vi "Dashboard Main.vi"() -> ()   [LabVIEW 2014]
uses:
  <vilib>/event_ctls.llb/eventvkey.ctl
  <vilib>/Utility/config.llb/NI_LVConfig.lvlib
  <vilib>/Rock Robotics/WPI/Dashboard/WPI_DashboardLogging Global.vi
  <vilib>/Utility/config.llb/Write Key (Boolean).vi
  <vilib>/Utility/config.llb/Write Key (String).vi
panel:
  out "Time":string
  out "Process?":bool
  in  "Listbox":i32(listbox)
  out "Progress":T1 {"Test Progress" scale=0.0..100.0}
  in  "Motor":cluster{"Value":dbl, "Enable":bool} {"Value" scale=-1.0..1.0 scale format="%#_3g"}
  in  "Test Slider":dbl(slide) scale=0.0..100.0 scale format="%#_3g"
  in  "On/Off":bool caption="Solenoid"
  in  "Test Name":u16(ring) items=["Select the test to run..."]
  in  "Rev/Fwd":cluster{"Forward":bool, "Reverse":bool}
  in  "Test Ring":u16(ring) items=["Monochrome", "Color"]
  in  "Test Tree":string(tree)
  in  "DB/String 9":string
  in  "DB/String 8":string
  in  "DB/String 7":string
  in  "DB/String 6":string
  in  "DB/String 5":string
  in  "DB/String 4":string
  in  "DB/String 3":string
  in  "DB/String 2":string
  in  "DB/String 1":string
  in  "DB/String 0":string
  in  "DB/Slider 0":dbl(slide) scale=0.0..5.0
  in  "DB/Slider 1":dbl(slide) scale=0.0..5.0
  in  "DB/Slider 2":dbl(slide) scale=0.0..5.0
  in  "DB/Slider 3":dbl(slide) scale=0.0..5.0
  out "DB/LED 3":bool
  out "DB/LED 2":bool
  out "DB/LED 1":bool
  out "DB/LED 0":bool
  in  "DB/Button 3":bool
  in  "DB/Button 2":bool
  in  "DB/Button 1":bool
  in  "DB/Button 0":bool caption="New Name"
  in  "TCP":refnum<k5>
  in  "Rec Mode":enum32{"Stop", "Record", "Playback"}(radio)
  in  "Vision":u16(ring) items=["Camera Off", "USB Camera SW", "USB Camera HW", "IP Camera"]
  out "Camera IP":string
  out "Image Message":string="Timeout in Camera Communications"
  in  "Dashboard Tab":T2(tab)
  out "Gyro":dbl(knob) scale=0.0..360.0
  out "JS1 Z 3":dbl(slide) scale=-1.0..1.0 scale format="%#_2e"
  out "JS1 Graph 3":cluster{"X":dbl, "Y":dbl}[](graph)
  out "JS1 Buttons 3":T3
  out "JS1 Z 2":dbl(slide) scale=-1.0..1.0 scale format="%#_2e"
  out "JS1 Graph 2":cluster{"X":dbl, "Y":dbl}[](graph)
  out "JS1 Buttons 2":T3
  in  "Dropdown":u8(ring) items=["Red 1", "Red 2", "Red 3", "Blue 1", "Blue 2", "Blue 3"]
  out "MotorChart R":cluster{"Numeric":dbl, "Numeric":dbl}(graph)
  out "MotorChart L":T4(graph)
  out "MotorSliders R":cluster{"MotorSlide1":dbl, "MotorSlide2":dbl} {"MotorSlide2" scale=-1.0..1.0 scale format="%#_2e"; "MotorSlide1" scale=-1.0..1.0 scale format="%#_2e"}
  out "MotorSliders L":T5 {"MotorSlide4 2" scale=0.0..14.0 scale format="%#_2e"; "MotorSlide2" scale=-1.0..1.0 scale format="%#_2e"; "MotorSlide1" scale=-1.0..1.0 scale format="%#_2e"}
  out "JS1 Z":dbl(slide) scale=-1.0..1.0 scale format="%#_2e"
  out "JS1 Graph":cluster{"X":dbl, "Y":dbl}[](graph)
  out "JS1 Buttons":T3
  out "Robot IP":string
  out "Dash Milliseconds Per Iteration":u32(knob) scale=250.0..500.0
  out "Dash Iterations Per Second":u32(knob)=4
  out "Main Milliseconds Per Iteration":u32(knob) scale=20.0..50.0
  out "CAN":T6 {"% Bus Utilization" format="%#_g%"}
  out "CAN BUS %":sgl(slide) scale=0.0..100.0
  out "CPU %":sgl(slide) scale=0.0..100.0
  out "RAM Usage":u32(slide) scale=0.0..100.0
  out "Storage":T7
  out "CPU Utilization":T8 {"CPU % ISR" format="%#_g%"; "CPU % Time Crit" format="%#_g%"; "CPU % Timed Str" format="%#_g%"; "CPU % High" format="%#_g%"; "CPU % Above" format="%#_g%"; "CPU % Normal" format="%#_g%"; "CPU % Low" format="%#_g%"}
  out "Main Iterations Per Second":u32(knob)=50
  in  "export stat":bool
  out "Stats":sgl[](graph)
  in  "clear stat":bool
  out "Tree":string(tree)
  out "Camera Image":T9(plugin-control)
  out "Boolean":bool
  # "Joysticks"
  # "SubStates"
  # "Drive & Battery"
  # "Encoders"
  # "Left"
  # "Front"
  # "Right"
  # "Battery"
  # "Chart of the below shown  data over time on next tab"
  # "Robot Metrics"
  # "Code Statistics"
  # "IPS"
  # "mSPI"
  # "IPS"
  # "mSPI"
  # "See the below driver station for\ngraphs of CPU%"
  # "Optimal Speeds (Statistics)\n\nMain mSPI = 20 ms\nMain IPS  = 50 iterations\n\nDash mSPI = 250 ms\nDash IPS  = 4 iterations\n\nKey\n\nmSPI - miliseconds per iteration\nIPS - iterations per second"
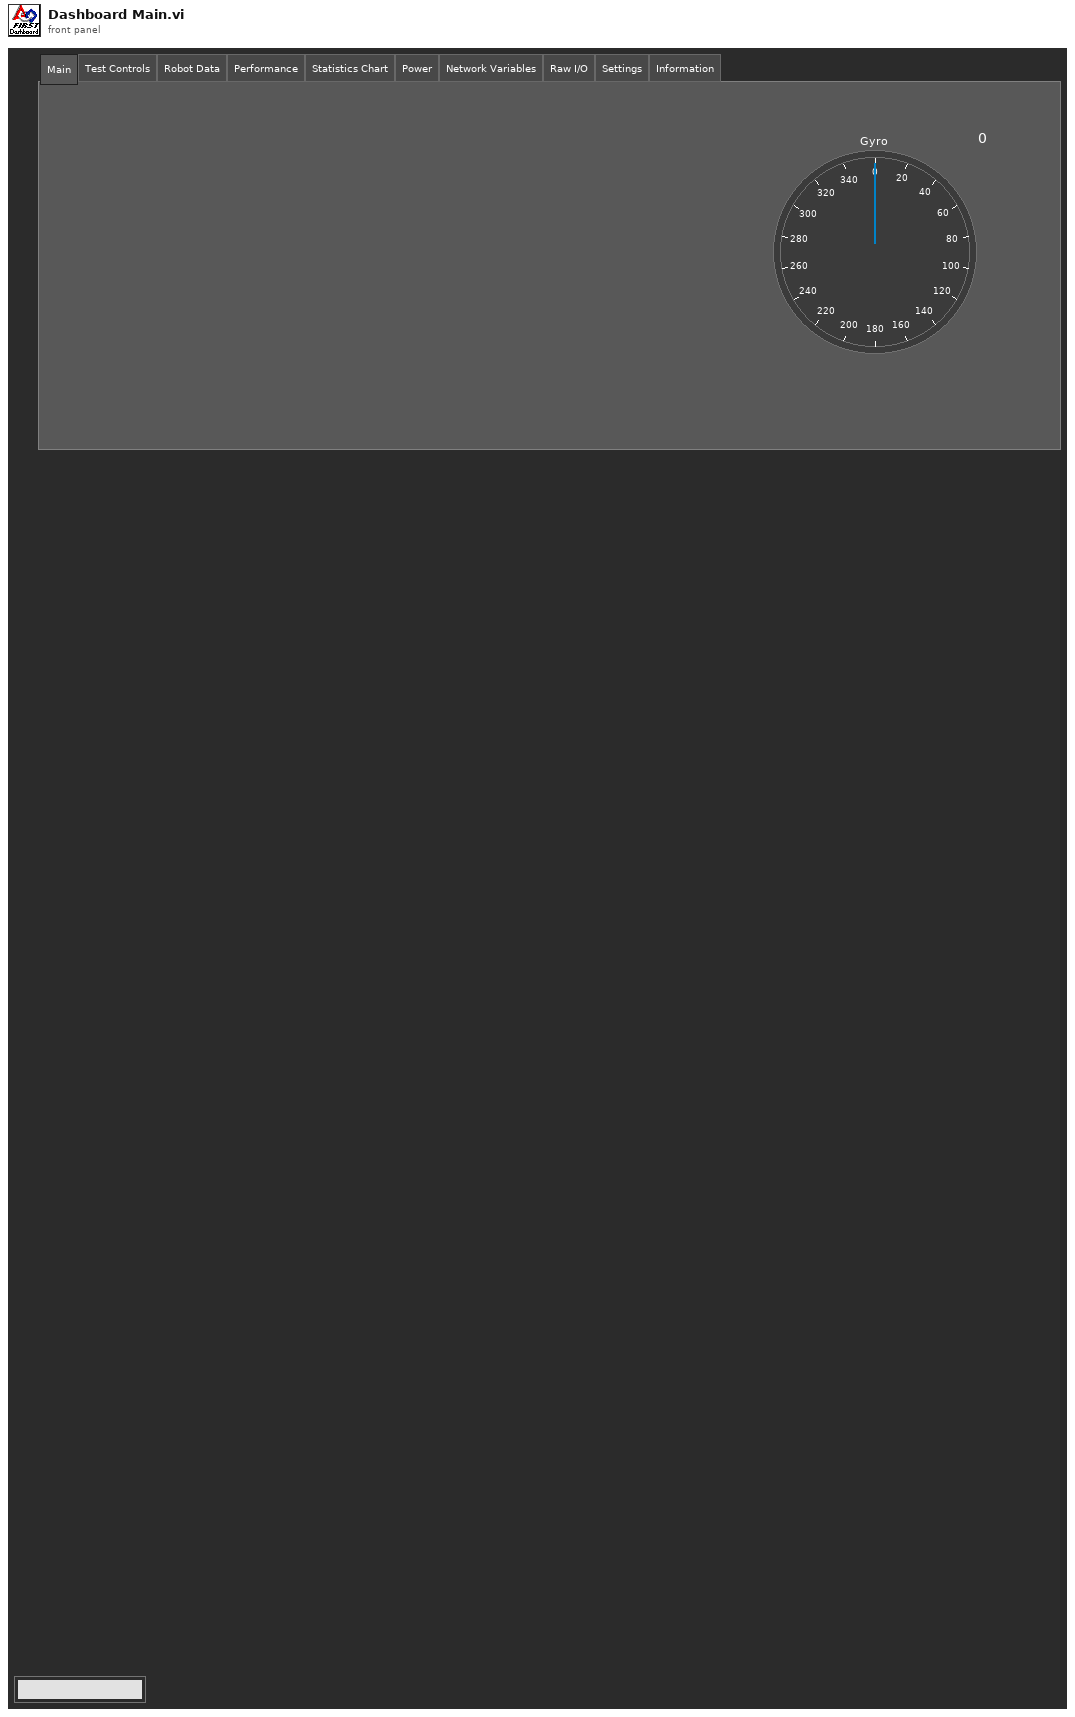
[diagram p1: front panel]
types:
  T1 = cluster{"Test Progress":u8, "Test Progress Text":string}
  T2 = enum32{"Main", "Test Controls", "Robot Data", "Performance", "Statistics Chart", "Power", "Network Variables", "Raw I/O", "Settings", "Information"}
  T3 = cluster{bool, bool, bool, bool, bool, bool, bool, bool, bool, bool, bool, bool}
  T4 = cluster{"Numeric":dbl, "Numeric":dbl, "Battery V":dbl}
  T5 = cluster{"MotorSlide1":dbl, "MotorSlide2":dbl, "MotorSlide4 2":dbl}
  T6 = cluster{"% Bus Utilization":sgl, "Bus Off Cnt":u32, "TX_FIFO Full Cnt":u32, "Receive Error Cnt":u8, "Transmit Error Cnt":u8}
  T7 = cluster{"Disk Free":u64, "RAM Block":u32, "RAM free":u32}
  T8 = cluster{"CPU % ISR":sgl, "CPU % Time Crit":sgl, "CPU % Timed Str":sgl, "CPU % High":sgl, "CPU % Above":sgl, "CPU % Normal":sgl, "CPU % Low":sgl}
  T9 = typedef "IMAQ Image.ctl" = refnum<image>
  T10 = enum32{"Drive", "Basic", "Custom", "Test", "Checklist", "Variables"}
  T11 = cluster{"Camera Image":refnum<vi>, "Dashboard Tab":refnum<vi>, "Boolean":refnum<vi>, "Vision":refnum<vi>, "Rec Mode":refnum<vi>, "Test Slider":refnum<vi>, "On/Off ":refnum<vi>, "Test Ring":refnum<vi>, "Rev/Fwd":refnum<vi>, "Test Name":refnum<vi>, "Motor":refnum<vi>, "Progress":refnum<vi>, "CheckList":refnum<vi>, "Tree":refnum<vi>, "Test Tree":refnum<vi>}
  T12 = cluster{"Error Strings":string, "Disable Counts":cluster{u16, u16}, "Rail Faults":cluster{u16, u16, u16}, "Robot IP":string, "DB Mode":u8, "Event Info":cluster{"Name":string, "Type":u8, "Number":u16, "Replay":u8}, "Camera Addr":string}
  T13 = cluster{"Storage":cluster{"Disk Free":u64, "RAM Block":u32, "RAM free":u32}, "CPU Utilization":cluster{"CPU % ISR":sgl, "CPU % Time Crit":sgl, "CPU % Timed Str":sgl, "CPU % High":sgl, "CPU % Above":sgl, "CPU % Normal":sgl, "CPU % Low":sgl}, "CAN":cluster{"% Bus Utilization":sgl, "Bus Off Cnt":u32, "TX_FIFO Full Cnt":u32, "Receive Error Cnt":u8, "Transmit Error Cnt":u8}, "HID":cluster{"HID Outputs":u32, "Rumble Low":u16, "Rumble High":u16}[]}
  T14 = cluster{"Status bits":cluster{"Test Mode":bool, "Autonomous":bool, "Enabled":bool, "Code Start":bool, "Brownout":bool, "Reserved 2":bool, "Reserved 3":bool, "E-Stop":bool}, "Code Trace":cluster{"Disabled":bool, "TeleOp":bool, "Auto":bool, "Test":bool}, "Controller Type":enum16{"unknown", "cRIO", "roboRio"}, "Code?":enum16{"unknown", "noCode", "code"}, "Battery V":dbl}
  T15 = cluster{"Control Bits":cluster{"TestMode":bool, "Autonomous":bool, "Enabled":bool, "FMS Present":bool, bool, bool, bool, "E-Stop":bool}, "Team Station ":u8, "Countdown":sgl, "Joystick Values":cluster{"Axes":dbl[], "Buttons":bool[], "POVs":i16[]}[]}
  T16 = enum8{"Tele-Op Disabled", "Tele-Op Enabled", "Auto Disabled", "Auto Enabled", "Test Disabled", "Test Enabled", "Disconnected", "No Code", "E-Stop"}
  T17 = cluster{"Axes":dbl[], "Buttons":bool[], "POVs":i16[]}[]
  T18 = cluster{"Axes":dbl[], "Buttons":bool[], "POVs":i16[]}
  T19 = cluster{"Buttons[0]":bool, "Buttons[1]":bool, "Buttons[2]":bool, "Buttons[3]":bool, "Buttons[4]":bool, "Buttons[5]":bool, "Buttons[6]":bool, "Buttons[7]":bool, "Buttons[8]":bool, "Buttons[9]":bool, "Buttons[10]":bool, "Buttons[11]":bool}
  T20 = typedef "Image Type" = u32
  T21 = typedef "WPI_CameraSettings Read MJPG.ctl" = cluster{"fps":i32, "compression":i32, "Image Size":T22}
  T22 = typedef "WPI_CameraImageSize.ctl" = enum16{"640x480", "320x240", "160x120", "Custom"}
  T23 = cluster{"Operation":enum16{"Update", "Clear"}, "Color Box":u32}[]
  T24 = typedef "eventvkey.ctl" = enum16{"ASCII", "Enter", "Return", "Shift", "Ctrl", "Alt", "Cmd", "Opt", "Caps", "NumLock", "Clear", "Break", "Up", "Down", "Left", "Right", "Insert", "Delete", "Home", "End", "PageUp", "PageDown", "Escape", "Help", "Pause", "ScrollLock", "F1", "F2", "F3", "F4", "F5", "F6", "F7", "F8", "F9", "F10", "F11", "F12", "F13", "F14", "F15", "F16", "F17", "F18", "F19", "F20", "F21", "F22", "F23", "F24", "Play", "VolumeUp", "VolumeDown", "Mute", "Two Byte Char"}
  T25 = cluster{"Image Size":bool, "Image Type":bool, "Pixel Value":bool, "ROI Information":bool, "Zoom Factor":bool}
  T26 = enum8{"Enabled", "Disabled", "Disabled and Grayed Out"}
  T27 = typedef "NI_LVConfig.lvlib/Config Data RefNum.ctl" = refnum<k1>
  T28 = cluster{"Operation":enum16{"Update", "Clear"}, "Color Box":u32}
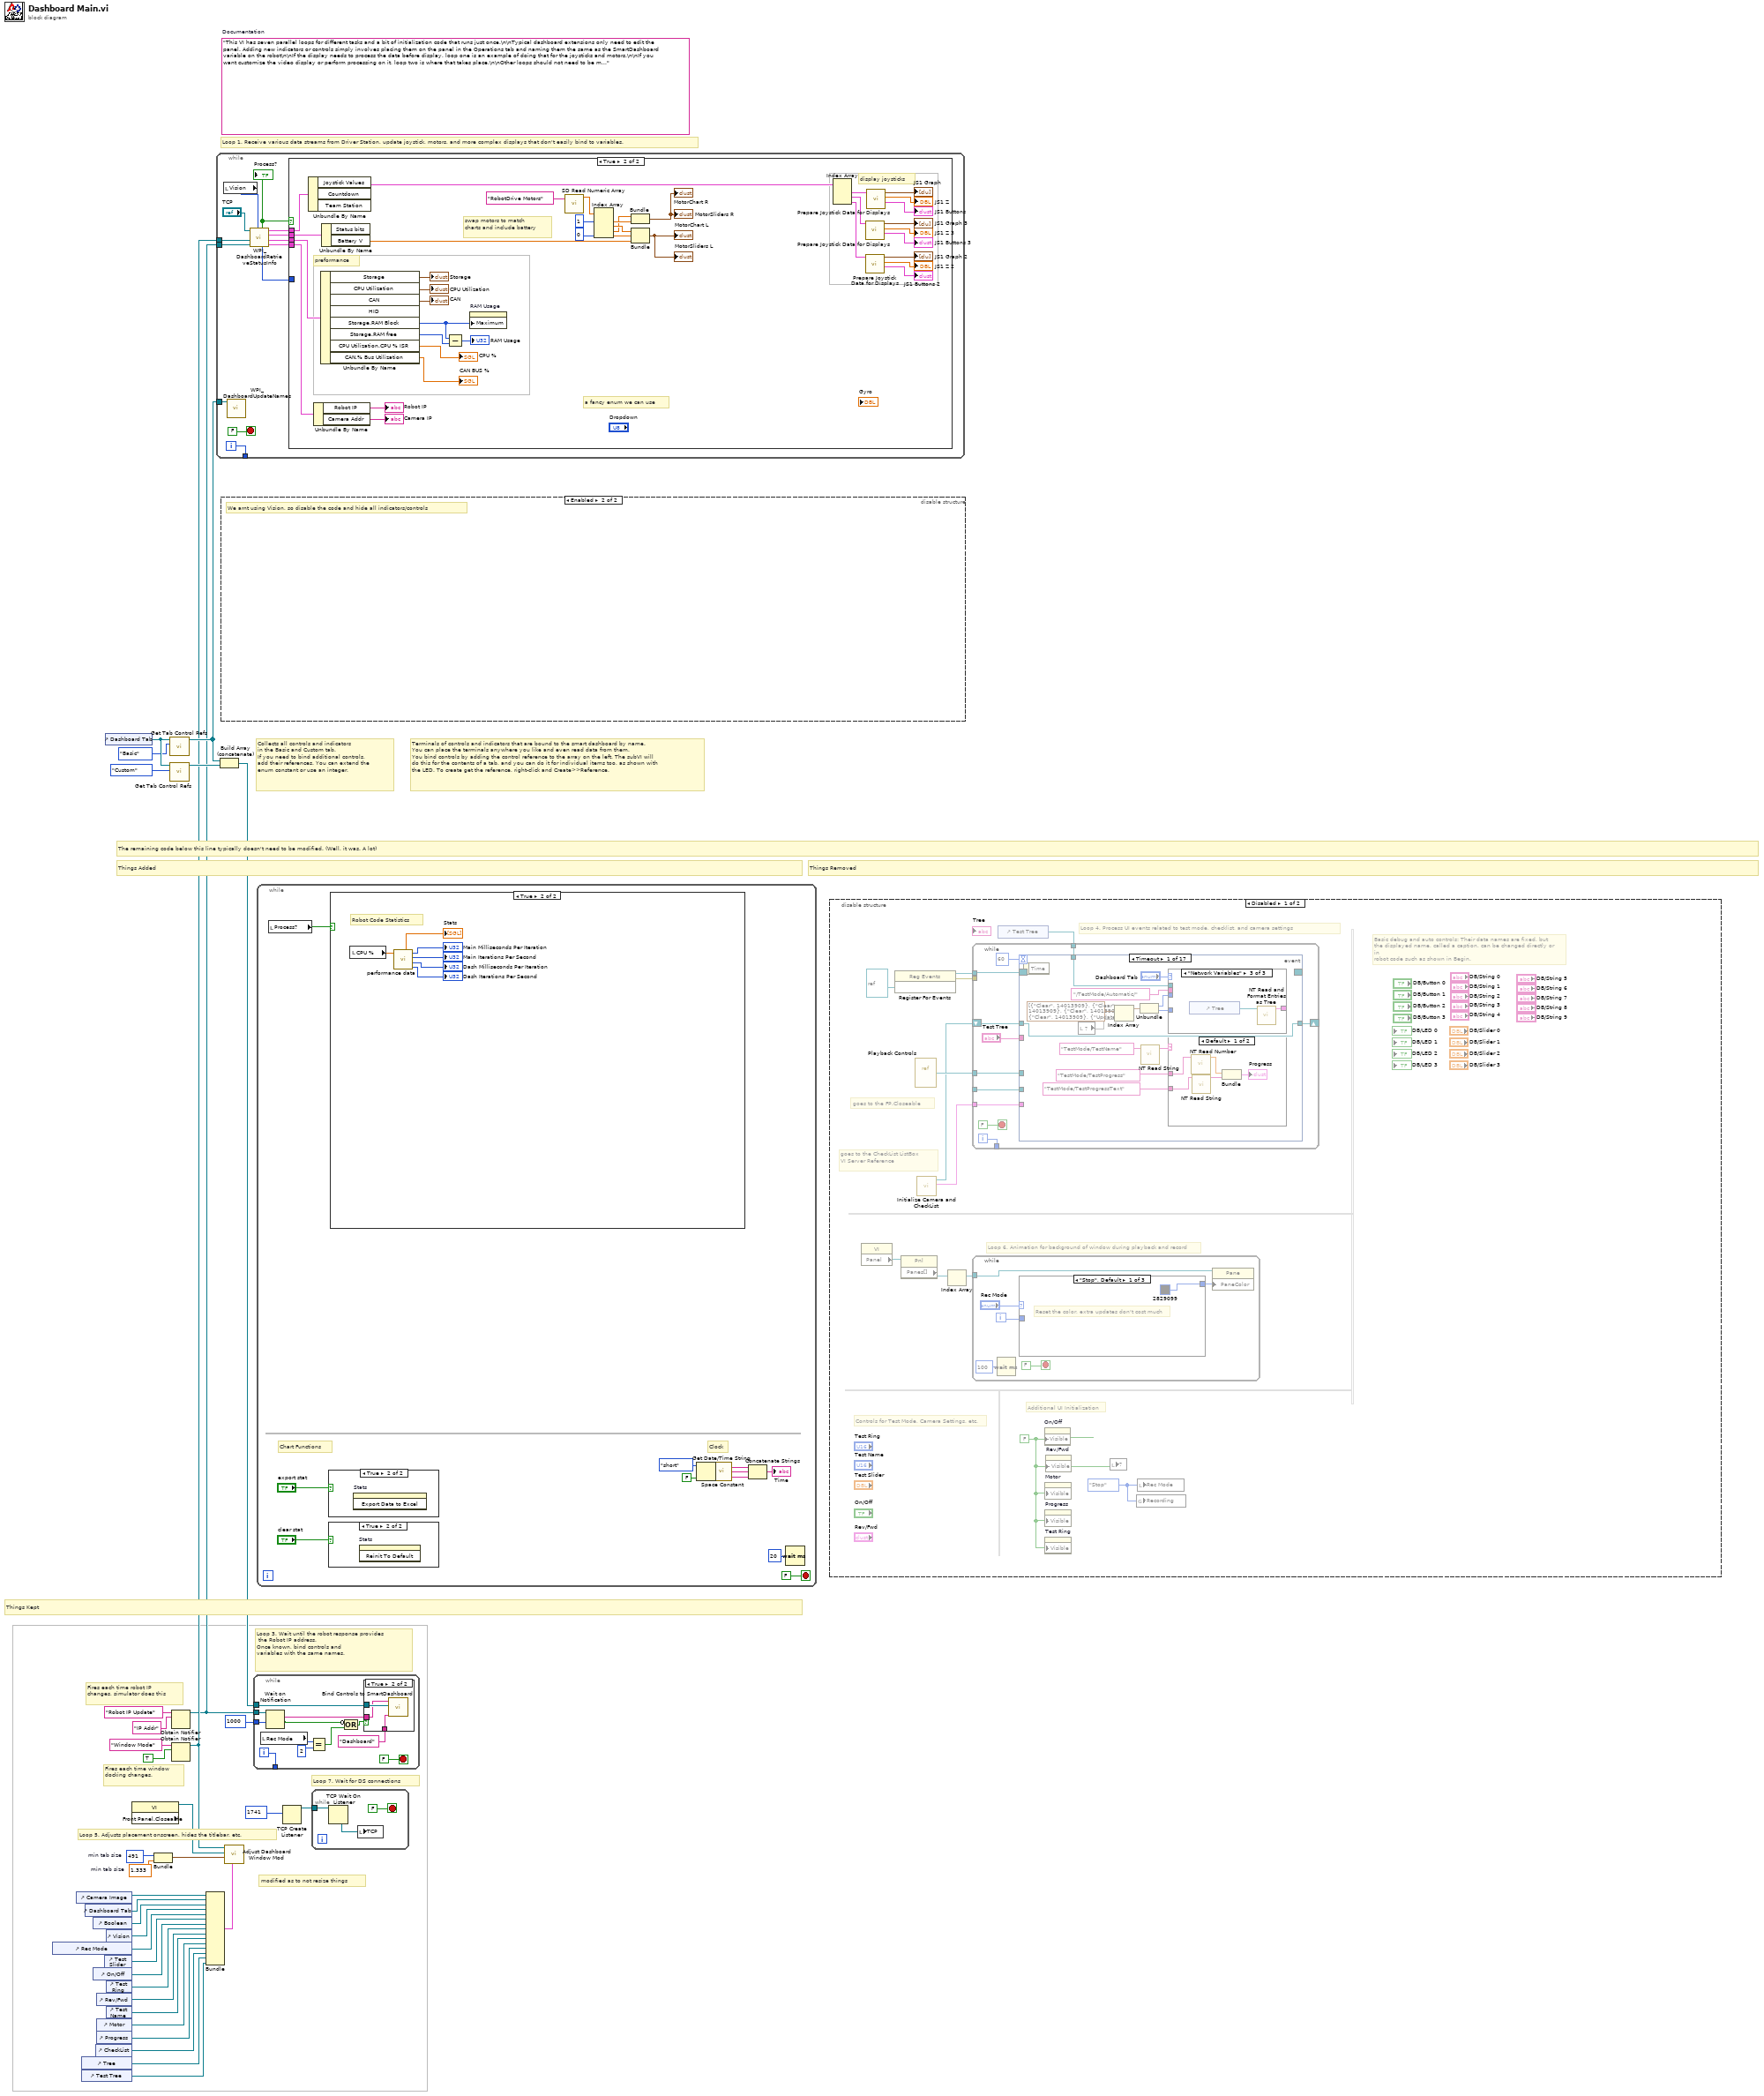
[diagram p0: block diagram]
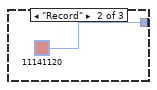
[diagram p5: hidden frame]
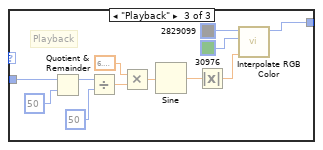
[diagram p6: hidden frame]
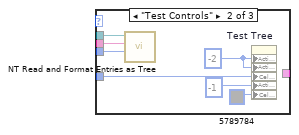
[diagram p8: hidden frame]
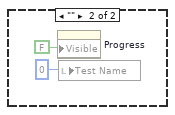
[diagram p9: hidden frame]
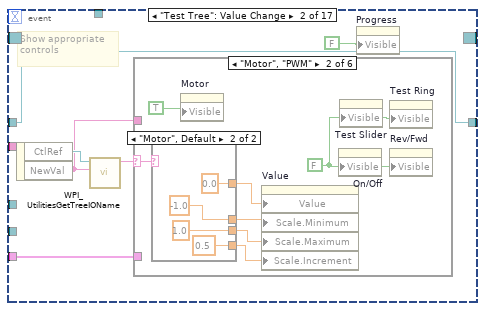
[diagram p10: hidden frame]
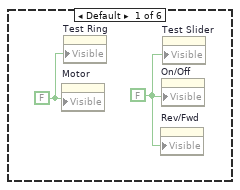
[diagram p11: hidden frame]
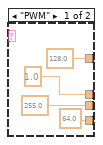
[diagram p12: hidden frame]
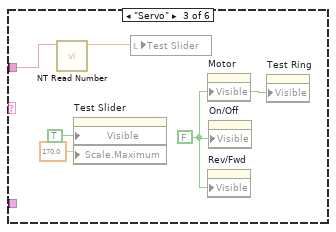
[diagram p13: hidden frame]
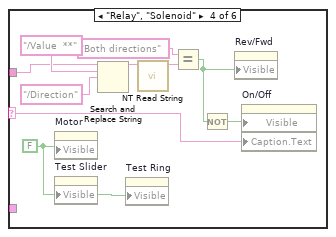
[diagram p14: hidden frame]
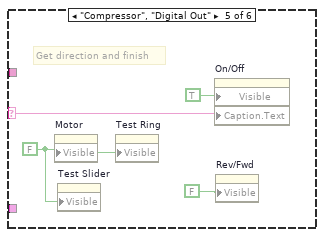
[diagram p15: hidden frame]
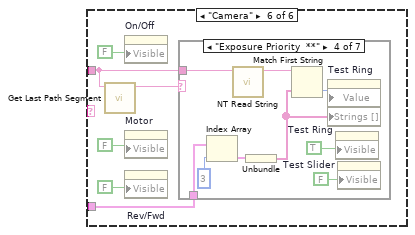
[diagram p16: hidden frame]
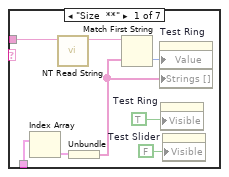
[diagram p17: hidden frame]
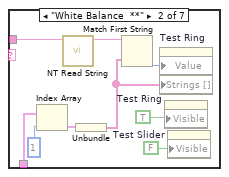
[diagram p18: hidden frame]
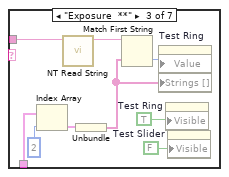
[diagram p19: hidden frame]
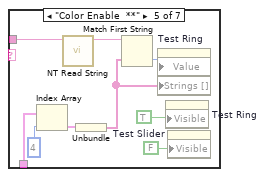
[diagram p20: hidden frame]
diagram:
  w24 = 491  # min tab size
  w23 = 1.333  # min tab size
  (unwired) "This VI has seven parallel loops for different tasks and a bit of initialization code that runs just once.\n\nTypical dashboard extensions only need to edit the panel. Adding new indicators or controls simply involves placing them on the panel in the Operations tab and naming them the same as the SmartDashboard variable on the robot\n\nIf the display needs to process the data before display, loop one is an example of doing that for the joysticks and motors.\n\nIf you want customize the video display or perform processing on it, loop two is where that takes place.\n\nOther loops should not need to be modified. They are pretty standard, and document the task they perform."  # Documentation
  # "modified as to not resize things"
  # "Things Kept"
  # "Things Added"
  # "Things Removed"
  # "Loop 7. Wait for DS connections"
  # "Fires each time robot IP\nchanges, simulator does this"
  # "Fires each time window\ndocking changes."
  # "Collects all controls and indicators\nin the Basic and Custom tab.\nIf you need to bind additional controls,\nadd their references. You can extend the\nenum constant or use an integer."
  # "The remaining code below this line typically doesn't need to be modified. (Well, it was. A lot)"
  # "Terminals of controls and indicators that are bound to the smart dashboard by name.\nYou can place the terminals anywhere you like and even read data from them.\nYou bind controls by adding the control reference to the array on the left. The subVI will\ndo this for the contents of a tab, and you can do it for individual items too, as shown with\nthe LED. To create get the reference, right-click and Create>>Reference."
  # "Loop 3. Wait until the robot response provides\n the Robot IP address.\nOnce known, bind controls and\nvariables with the same names."
  # "Loop 5. Adjusts placement onscreen, hides the titlebar, etc."
  # "Loop 1. Receive various data streams from Driver Station, update joystick, motors, and more complex displays that don't easily bind to variables."
  n1 = control-ref of="Rec Mode"() -> (w15:refnum<vi>)
  n2 = control-ref of="Camera Image"() -> (w27:refnum<vi>)
  n3 = control-ref of="Tree"() -> (w19:refnum<vi>)
  n4 = control-ref of="Test Tree"() -> (w18:refnum<vi>)
  n5 = control-ref of="Dashboard Tab"() -> (w26:refnum<vi>)
  n6 = control-ref of="Boolean"() -> (w22:refnum<vi>)
  n7 = control-ref of="On/Off"() -> (w13:refnum<vi>)
  n8 = control-ref of="CheckList"() -> (w6:refnum<vi>)
  n9 = control-ref of="Rev/Fwd"() -> (w11:refnum<vi>)
  n10 = control-ref of="Motor"() -> (w16:refnum<vi>)
  n11 = control-ref of="Progress"() -> (w10:refnum<vi>)
  n12 = control-ref of="Test Slider"() -> (w14:refnum<vi>)
  n13 = control-ref of="Dashboard Tab"() -> (w30:refnum<vi>)
  n14 = control-ref of="Vision"() -> (w25:refnum<vi>)
  n15 = control-ref of="Test Ring"() -> (w12:refnum<vi>)
  n16 = control-ref of="Test Name"() -> (w17:refnum<vi>)
  n17 = property class="VI" props=["Front Panel.Closeable"]() -> (reference out=w3:refnum<vi>)  [unwired: 2 in, 2 out]
  n18 = Bundle("min tab size"=w24, "min tab size"=w23) -> (w4:cluster{"min tab size":i32, "min tab size":dbl})  [unwired: 1 in]
  n19 = call <vilib>:"Get Tab Control Refs.vi"("Page Index"=T10."Basic" ("Dashboard Tab"), "TabControl in"=w30) -> ("ControlsOnPage"=w9:refnum<vi>[])  [unwired: 9 in]
  n20 = call <vilib>:"Get Tab Control Refs.vi"("Page Index"=T10."Custom" ("Dashboard Tab"), "TabControl in"=w30) -> ("ControlsOnPage"=w29:refnum<vi>[])  [unwired: 9 in]
  n21 = Obtain Notifier(name (unnamed)="Robot IP Update", notification data type="IP Addr" ("name (unnamed)")) -> (notifier out=w1:refnum<notifier>)  [unwired: 2 in, 2 out]
  n22 = Obtain Notifier(name (unnamed)="Window Mode", notification data type=TRUE) -> (notifier out=w2:refnum<notifier>)  [unwired: 2 in, 2 out]
  n23 = Bundle("Camera Image"=w27, "Dashboard Tab"=w26, "Boolean"=w22, "Vision"=w25, "Rec Mode"=w15, "Test Slider"=w14, "On/Off"=w13, "Test Ring"=w12, "Rev/Fwd"=w11, "Test Name"=w17, "Motor"=w16, "Progress"=w10, "CheckList"=w6, "Tree"=w19, "Test Tree"=w18) -> (w5:T11)  [unwired: 1 in]
  n24 = while {
    tunnel: [w47] -> _
    tunnel: w1 -> [w41]
    tunnel: w9 -> [w40]
    tunnel: w2 -> [w36]
    i -> [w47]
    stop <- FALSE stop-if-true
    n25 = local read "Vision"() -> (w38:u16)
    n26 = call <vilib>:"WPI_DashboardUpdateNames.vi"("Controls on Tab"=w40) -> ()  [unwired: 11 in]
    n27 = call <vilib>:"WPI_DashboardRetrieveStatusInfo.vi"("Vision"=w38, "Binding Refnum"=w41, "Window Mode Notifier"=w36, "TCP Cnx"="TCP") -> ("Power and Errors"=w42:T12, "Robot Metrics"=w45:T13, "Status Info"=w46:T14, "Control Info"=w43:T15, "Robot Mode"=w39:T16, "Process?"=w44:bool)  [unwired: 2 in]
    "Process?" <- w44
    n28 = case shown="True" w44 {
      tunnel: w46 -> [_ w86]
      tunnel: w45 -> [_ w85]
      tunnel: w43 -> [_ w84]
      tunnel: w42 -> [_ w83]
      tunnel: w39 -> [_ _]
      frame False {
      }
      frame True {
        # "preformance"
        # "display joysticks"
        # "a fancy enum we can use"
        # "swap motors to match\ncharts and include battery"
        n29 = Unbundle By Name(w84) -> ("Joystick Values"=w73:T17)  [unwired: 2 out]
        n30 = Unbundle By Name(w83) -> ("Robot IP"=→"Robot IP":string, "Camera Addr"=→"Camera IP":string)
        n31 = Unbundle By Name(w85) -> ("Storage"=→"Storage":T7, "CPU Utilization"=→"CPU Utilization":T8, "CAN"=→"CAN":T6, "Storage.RAM Block"=w52:u32, "Storage.RAM free"=w51:u32, "CPU Utilization.CPU % ISR"=→"CPU %":sgl, "CAN.% Bus Utilization"=→"CAN BUS %":sgl)  [unwired: 1 out]
        n32 = Unbundle By Name(w86) -> ("Battery V"=w74:dbl)  [unwired: 1 out]
        n33 = Subtract(x=w52, y=w51) -> (x-y=→"RAM Usage":u32)
        n34 = property on="RAM Usage" class="Slide (strict)"("Maximum"=w52) -> ()  [unwired: 2 in, 2 out]
        n35 = call <vilib>:"SD Read Numeric Array.vi"("Name"="RobotDrive Motors") -> ("Numeric Array"=w76:dbl[])  [unwired: 8 in, 2 out]
        n36 = Index Array(array=w76, index #1=1, index #4=0) -> (element #1=w78:dbl, element #2=w79:dbl, element #3=w77:dbl, element #4=w82:dbl)  [unwired: 2 in]
        n37 = Bundle("Numeric"=w77, "Numeric"=w78) -> (→"MotorSliders R" →"MotorChart R":cluster{"Numeric":dbl, "Numeric":dbl})  [unwired: 1 in]
        n38 = Bundle("Numeric"=w79, "Numeric"=w82, "Battery V"=w74) -> (→"MotorSliders L" →"MotorChart L":T4)  [unwired: 1 in]
        n39 = Index Array(array=w73) -> (element #1=w72:T18, element #2=w70:T18, element #3=w66:T18)  [unwired: 3 in]
        n40 = call "Prepare Joystick Data for Displays.vi"("Joystick Values"=w70) -> ("Buttons"=→"JS1 Buttons 3":T19, "Z Axis"=→"JS1 Z 3":dbl, "Cartesian Data"=→"JS1 Graph 3":cluster{"X axis":dbl, "X axis":dbl}[])  [unwired: 8 in]
        n41 = call "Prepare Joystick Data for Displays.vi"("Joystick Values"=w66) -> ("Buttons"=→"JS1 Buttons 2":T19, "Z Axis"=→"JS1 Z 2":dbl, "Cartesian Data"=→"JS1 Graph 2":cluster{"X axis":dbl, "X axis":dbl}[])  [unwired: 8 in]
        n42 = call "Prepare Joystick Data for Displays.vi"("Joystick Values"=w72) -> ("Buttons"=→"JS1 Buttons":T19, "Z Axis"=→"JS1 Z":dbl, "Cartesian Data"=→"JS1 Graph":cluster{"X axis":dbl, "X axis":dbl}[])  [unwired: 8 in]
      }
    }
  }
  n43 = Build Array (concatenate)(w9, w29) -> (w28:refnum<vi>[])
  n44 = disable-structure shown="Enabled" {
    frame Disabled {
      w89 = T20 4 items=["Grayscale (U8)", "Grayscale (I16)", "Grayscale (SGL)", "Complex (CSG)", "RGB (U32)", "HSL (U32)", "RGB (U64)"] ("Image Type")
      # "unwired controls/indicators from below that orange line :P"
      # "Loop 2. Receive camera images from Robot, update Mbps, fps, and do any processing or display"
      n45 = call "IMAQ Create"("Image Name"="Dashboard Image", "Image Type"=w89) -> ("New Image"=w87:T9, "error out"=w88:errorcluster)  [unwired: 2 in, 1 out]
      n46 = while {
        tunnel: w87 -> [w99]
        tunnel: w88 -> [_]
        tunnel: [w100] -> _
        i -> [w100]
        stop <- FALSE stop-if-true
        # "Optionally read the DB image,\nlog, or retrieve images from a\nlogged match"
        n47 = local read "Rec Mode"() -> (w93:enum32{"Stop", "Record", "Playback"})
        n48 = local read "Camera IP"() -> (w91:string)
        n49 = call <vilib>:"WPI_CameraRead MJPG for Dashboard.vi"("Rec Mode"=w93, "Camera IP"=w91, "Camera Mode"="Vision", "Refnum in"=w99) -> ("Active"=w97:bool, "Refnum out"=w98:T9, "FPS"=w96:dbl, "Bandwidth (Mbps)"=w95:dbl, "Camera Settings"=w94:T21)  [unwired: 3 in]
        n50 = case shown="True" w97 {
          tunnel: w98 -> [_ w106]
          tunnel: w95 -> [_ w105]
          tunnel: w96 -> [_ w103]
          frame False {
            # "Sleep for 500ms"
            n51 = Wait Until Next ms Multiple(millisecond multiple=u32 500) -> ()  [unwired: 1 out]
          }
          frame True {
            # "Here is where you would annotate,\npossibly process, and display the image"
            # "Update Mbps LED"
            n52 = call "IMAQ Clear Overlay"("Image"=w106) -> ("error out"=w109:errorcluster, "Image Out"=→"Camera Image":T9)  [unwired: 2 in, 7 out]
            n53 = case shown="4, 5" w105 {
              tunnel: [u32 6618880 ("Color Box") u32 16776722 ("Color Box") u32 16716800 ("Color Box")] -> w107
              frame Default {
              }
              frame 4, 5 {
              }
              frame 6.. {
              }
            }
            n54 = Unbundle By Name(w109) -> ("status"=w110:bool)
            n55 = Bundle("Color Box"=w107, "Color Box"=w107) -> (w108:cluster{"Color Box":u32, "Color Box":u32})  [unwired: 1 out]
            n56 = property on="Image Message" class="Str"("Visible"=w110) -> ()  [unwired: 2 in, 2 out]
            n57 = Build Array(w108) -> ()  [unwired: 1 out]
          }
        }
      }
    }
    frame Enabled {
      # "We arnt using Vision, so disable the code and hide all indicators/controls"
    }
  }
  n58 = call "Adjust Dashboard Window Mod.vi"("Sizing Refnums"=w5, "Size Constraints"=w4, "VI"=w3, "Notifier in"=w2) -> ()  [unwired: 8 in]
  n59 = while {
    tunnel: w28 -> [w125]
    tunnel: w1 -> [w123]
    tunnel: [w121] -> _
    tunnel: u32 1000 ("milliseconds to wait") -> [w120]
    i -> [w121]
    stop <- FALSE stop-if-true
    n60 = local read "Rec Mode"() -> (w116:enum32{"Stop", "Record", "Playback"})
    n61 = Wait on Notification(notifier=w123, timeout in ms (-1)=w120) -> (notification=w122:string, timed out?=w118:bool)  [unwired: 2 in, 2 out]
    n62 = Equal?(x=w116, y=u16 2 ("Rec Mode")) -> (x = y?=w117:bool)
    n63 = Compound Arithmetic op=OR(invert w118, w117) -> (w119:bool)
    n64 = case shown="True" w119 {
      tunnel: w125 -> [_ w128]
      tunnel: w122 -> [_ w127]
      tunnel: "Dashboard" -> [_ w126]
      frame False {
      }
      frame True {
        n65 = call <vilib>:"Bind Controls to SmartDashboard.vi"("Client Name"=w126, "Bound Control Refs"=w128, "Server IP Address"=w127) -> ()  [unwired: 9 in]
      }
    }
  }
  n66 = while {
    stop <- FALSE stop-if-true
    # "Clock"
    # "Chart Functions"
    n67 = local read "Process?"() -> (w139:bool)
    n68 = case shown="True" "export stat" {
      frame False {
      }
      frame True {
        n69 = invoke on="Stats" class="WFChart (strict)" method="Export Data to Excel"() -> ()  [unwired: 3 in, 3 out]
      }
    }
    n70 = case shown="True" "clear stat" {
      frame False {
      }
      frame True {
        n71 = invoke on="Stats" class="WFChart (strict)" method="Reinit To Default"() -> ()  [unwired: 3 in, 3 out]
      }
    }
    n72 = case shown="True" w139 {
      frame False {
      }
      frame True {
        # "Robot Code Statistics"
        n73 = local read "CPU %"() -> (w144:sgl)
        n74 = call "performance data.vi"("CPU %"=w144) -> ("Dash IPS"=→"Dash Iterations Per Second":u32, "Dash mSPI"=→"Dash Milliseconds Per Iteration":u32, "Main IPS"=→"Main Iterations Per Second":u32, "Main mSPI"=→"Main Milliseconds Per Iteration":u32, "stats"=→"Stats":sgl[])  [unwired: 6 in]
      }
    }
    n75 = Get Date/Time String(date format (0)=enum16{"short", "long", "abbreviated"}."short", want seconds? (F)=FALSE) -> (date string=w131:string, time string=w132:string)  [unwired: 1 in]
    n76 = call <vilib>:"Space Constant.vi"() -> ("String"=w133:string)
    n77 = Concatenate Strings(w131, w133, w132) -> (→"Time":string)
    n78 = Wait (ms)(milliseconds to wait=u32 20) -> ()  [unwired: 1 out]
  }
  n79 = TCP Create Listener(10:u16 1741 ("timeout ms (25000)")) -> (3:w7:refnum<k5>)  [unwired: 4 in, 2 out]
  n80 = while {
    tunnel: w7 -> [w147]
    stop <- FALSE stop-if-true
    n81 = TCP Wait On Listener(11:w147) -> (4:w146:refnum<k5>)  [unwired: 3 in, 4 out]
    n82 = local write "TCP"(w146) -> ()
  }
  n83 = disable-structure shown="Disabled" {
    frame Disabled {
      w149 = enum32{"Stop", "Record", "Playback"}."Stop" ("Rec Mode")
      w150 = FALSE ("Visible")
      # "Basic debug and auto controls: Their data names are fixed, but\nthe displayed name, called a caption, can be changed directly or in\nrobot code such as shown in Begin."
      # "Additional UI Initialization"
      # "Controls for Test Mode, Camera Settings, etc."
      # "Loop 6. Animation for background of window during playback and record"
      # "goes to the CheckList ListBox\nVI Server Reference"
      # "goes to the FP.Closeable"
      # "Loop 4. Process UI events related to test mode, checklist, and camera settings"
      n84 = property class="VI"() -> ("Panel"=w152:refnum<vi>)  [unwired: 2 in, 2 out]
      n85 = register-events(refnum<vi> refnum) -> (reference out=w159:refnum<event-registration>, error out=w160:errorcluster)  [unwired: 2 in]
      n86 = property class="Pnl"(reference=w152) -> ("Panes[]"=w151:refnum<vi>[])  [unwired: 1 in, 2 out]
      n87 = vi-ref "Playback Controls.vi"() -> (w158:refnum<vi>)
      n88 = call "Initialize Camera and CheckList.vi"() -> ("Cluster"=w155:cluster{"value":i32, "value":i32, "index":i32}, "Array"=w154:cluster{string[]}[], "File Refnum"=w156:T27, "ListBox in"=w163:refnum<vi>)  [unwired: 8 in]
      n89 = Index Array(array=w151) -> (element=w153:refnum<vi>)  [unwired: 1 in]
      n90 = while {
        tunnel: w153 -> [w165]
        i -> [w168]
        stop <- FALSE stop-if-true
        n91 = Wait (ms)(milliseconds to wait=u32 100) -> ()  [unwired: 1 out]
        n92 = case shown="\"Stop\", Default" "Rec Mode" {
          tunnel: w168 -> [_ _ w183]
          tunnel: [u32 2829099 ("Base Color") u32 11141120 ("Target Color") w172] -> w164
          frame "Stop", Default {
            # "Reset the color, extra updates don't cost much"
          }
          frame "Record" {
          }
          frame "Playback" {
            # "Playback"
            n93 = Quotient & Remainder(x=w183, y=u32 50 ("milliseconds to wait")) -> (x-y*floor(x/y)=w179:u32)  [unwired: 1 out]
            n94 = Divide(x=w179, y=u32 50 ("milliseconds to wait")) -> (x/y=w176:dbl)
            n95 = Multiply(x=6.283185307179586, y=w176) -> (x*y=w181:dbl)
            n96 = Sine(x=w181) -> (sin(x)=w180:dbl)
            n97 = Absolute Value(x=w180) -> (abs(x)=w173:dbl)
            n98 = call "Interpolate RGB Color.vi"("Proportion"=w173, "Target Color"=u32 30976, "Base Color"=u32 2829099) -> ("Result Color"=w172:u32)  [unwired: 8 in]
          }
        }
        n99 = property class="Pane"(reference=w165, "PaneColor"=w164) -> ()  [unwired: 1 in, 2 out]
      }
      n100 = control-ref of="Test Tree"() -> (w157:refnum<vi>)
      n101 = while {
        tunnel: w154 -> [w191]
        shift-right: [w190] -> _
        shift-left: w156 -> [w189]
        tunnel: [w188] -> _
        tunnel: w157 -> [w187]
        tunnel: w158 -> [w186]
        tunnel: w159 -> [w185]
        tunnel: w160 -> [_]
        tunnel: [w184] -> w162
        i -> [w188]
        stop <- FALSE stop-if-true
        n102 = event shown="[0] Timeout" {
          selector: w185 -> [_ _ _ _ _ _ _ _ _ _ _ _ _ _ _ _ _]
          dyn-events: [_ _ _ _ _ _ _ _ _ _ _ _ _ w427 _ _ _] -> _
          timeout: u32 60 ("milliseconds to wait") -> [_ _ _ _ _ _ _ _ _ _ _ _ _ _ _ _ _]
          tunnel: w187 -> [w203 _ _ _ _ _ _ _ _ _ _ _ _ _ _ _ _]
          tunnel: "Test Tree" -> [_ _ _ _ _ _ _ _ w396 w404 w406 w410 w418 _ _ _ _]
          tunnel: w191 -> [_ w225 _ _ _ _ w362 w391 _ _ _ _ _ _ _ _ _]
          tunnel: [w199 w224 w323 w328 w336 w348 w361 w384 w395 w402 w405 w409 w417 w429 w443 w444 w454] -> w190
          tunnel: w189 -> [w199 w224 w323 w328 w336 w348 w360 w384 w395 w402 w405 w409 w417 w429 w443 w444 w454]
          tunnel: w186 -> [_ _ _ _ _ _ _ _ _ _ _ _ _ w430 _ w447 _]
          tunnel: w184 -> [_ _ _ _ _ _ _ _ _ _ _ _ _ w425 _ _ _]
          event Timeout {
            n103 = event-data() -> ()  [unwired: 1 in, 1 out]
            n104 = local read item#-1() -> (w202)
            n105 = Index Array(array=T23 [{"Operation"=enum."Clear", "Color Box"=14013909}, {"Operation"=enum."Clear", "Color Box"=14013909}, {"Operation"=enum."Clear", "Color Box"=14013909}, {"Operation"=enum."Clear", "Color Box"=14013909}, {"Operation"=enum."Update", "Color Box"=14013909}, {"Operation"=enum."Update", "Color Box"=16777215}, {"Operation"=enum."Clear", "Color Box"=14013909}, {"Operation"=enum."Clear", "Color Box"=14013909}, {"Operation"=enum."Clear", "Color Box"=14013909}], index=w202) -> (element=w197:T28)
            n106 = Unbundle(w197) -> ("Operation"=w196:enum16{"Update", "Clear"}, "Color Box"=w195:u32)
            n107 = call <vilib>:"NT Read String.vi"("Name"="TestMode/TestName") -> ("String"=w206:string)  [unwired: 9 in, 1 out]
            n108 = case shown="\"Network Variables\"" "Dashboard Tab" {
              tunnel: w203 -> [_ w214 _]
              tunnel: "/TestMode/Automatic/" ("Name Pattern") -> [_ w213 _]
              tunnel: w196 -> [_ w212 _]
              tunnel: [_ _ w216] -> _
              tunnel: w195 -> [_ w208 _]
              frame "Robot Data", Default {
              }
              frame "Test Controls" {
                w211 = -2 ("Active Item:Row Number")
                n109 = call <vilib>:"NT Read and Format Entries as Tree.vi"("Operation"=w212, "Name Pattern"=w213, "Tree Refnum"=w214) -> ()  [unwired: 7 in, 2 out]
                n110 = property on="Test Tree" class="Tree (strict)"("Active Item Row Number"=w211, "ActiveColNum"=w211, "CellBG"=w208, "Active Item Row Number"=-1 ("Active Item:Row Number"), "CellBG"=u32 5789784 ("Color Box")) -> ()  [unwired: 2 in, 2 out]
              }
              frame "Network Variables" {
                n111 = control-ref of="Tree"() -> (w215:refnum<vi>)
                n112 = call <vilib>:"NT Read and Format Entries as Tree.vi"("Tree Refnum"=w215) -> ("Formatted Strings"=w216:cluster{"Name":string, "Value":string}[])  [unwired: 9 in, 1 out]
              }
            }
            n113 = case shown="Default" w206 {
              tunnel: "TestMode/TestProgress" ("Name") -> [w218 _]
              tunnel: "TestMode/TestProgressText" ("Name") -> [w217 _]
              frame Default {
                n114 = call <vilib>:"NT Read Number.vi"("Name"=w218) -> ("Numeric"=w219:dbl)  [unwired: 9 in, 1 out]
                n115 = call <vilib>:"NT Read String.vi"("Name"=w217) -> ("String"=w220:string)  [unwired: 9 in, 1 out]
                n116 = Bundle("Numeric"=w219, "String"=w220) -> (→"Progress":cluster{"Numeric":dbl, "String":string})  [unwired: 1 in]
              }
              frame "" {
                n117 = property on="Progress" class="Clust (strict)"("Visible"=FALSE) -> ()  [unwired: 2 in, 2 out]
                n118 = local write "Test Name"(u16 0) -> ()
              }
            }
          }
          event "Test Tree": Value Change {
            # "Show appropriate\ncontrols"
            n119 = event-data() -> ("CtlRef"=w228:refnum<vi>, "NewVal"=w226:string)  [unwired: 1 in]
            n120 = call <vilib>:"WPI_UtilitiesGetTreeIOName.vi"("NewVal"=w226, "TreeControl in"=w228) -> ("I/O Name"=w229:string)  [unwired: 9 in]
            n121 = case shown="\"Motor\", \"PWM\"" w229 {
              selector: w229 -> [_ w236 _ w254 w263 _]
              tunnel: w226 -> [_ _ w251 w253 _ w270]
              tunnel: w225 -> [_ _ _ _ _ w269]
              frame Default {
                w231 = FALSE ("Visible")
                w230 = FALSE ("Visible")
                n122 = property on="Motor" class="Clust (strict)"("Visible"=w230) -> ()  [unwired: 2 in, 2 out]
                n123 = property on="Test Ring" class="Ring (strict)"("Visible"=w230) -> ()  [unwired: 2 in, 2 out]
                n124 = property on="Rev/Fwd" class="Clust (strict)"("Visible"=w231) -> ()  [unwired: 2 in, 2 out]
                n125 = property on="On/Off" class="Bool (strict)"("Visible"=w231) -> ()  [unwired: 2 in, 2 out]
                n126 = property on="Test Slider" class="Slide (strict)"("Visible"=w231) -> ()  [unwired: 2 in, 2 out]
              }
              frame "Motor", "PWM" {
                w237 = FALSE ("Visible")
                n127 = case shown="\"Motor\", Default" w236 {
                  tunnel: [1.0 ("Value") -1.0 ("Value")] -> w235
                  tunnel: [255.0 ("Value") 1.0 ("Value")] -> w234
                  tunnel: [128.0 ("Value") 0.0 ("Value")] -> w233
                  tunnel: [64.0 ("Value") 0.5 ("Value")] -> w232
                  frame "PWM" {
                  }
                  frame "Motor", Default {
                  }
                }
                n128 = property on="Motor" class="Clust (strict)"("Visible"=TRUE) -> ()  [unwired: 2 in, 2 out]
                n129 = property on="Value" class="Slide (strict)"("Value"=w233, "Scale.Minimum"=w235, "Scale.Maximum"=w234, "Scale.Increment"=w232) -> ()  [unwired: 2 in, 2 out]
                n130 = property on="On/Off" class="Bool (strict)"("Visible"=w237) -> ()  [unwired: 2 in, 2 out]
                n131 = property on="Test Slider" class="Slide (strict)"("Visible"=w237) -> ()  [unwired: 2 in, 2 out]
                n132 = property on="Test Ring" class="Ring (strict)"("Visible"=w237) -> ()  [unwired: 2 in, 2 out]
                n133 = property on="Rev/Fwd" class="Clust (strict)"("Visible"=w237) -> ()  [unwired: 2 in, 2 out]
              }
              frame "Servo" {
                w249 = FALSE ("Visible")
                n134 = call <vilib>:"NT Read Number.vi"("Name"=w251) -> ("Numeric"=w250:dbl)  [unwired: 9 in, 1 out]
                n135 = property on="Test Slider" class="Slide (strict)"("Visible"=TRUE, "Scale.Maximum"=170.0 ("Scale.Range:Maximum")) -> ()  [unwired: 2 in, 2 out]
                n136 = local write "Test Slider"(w250) -> ()
                n137 = property on="Motor" class="Clust (strict)"("Visible"=w249) -> ()  [unwired: 2 in, 2 out]
                n138 = property on="Rev/Fwd" class="Clust (strict)"("Visible"=w249) -> ()  [unwired: 2 in, 2 out]
                n139 = property on="On/Off" class="Bool (strict)"("Visible"=w249) -> ()  [unwired: 2 in, 2 out]
                n140 = property on="Test Ring" class="Ring (strict)"("Visible"=w249) -> ()  [unwired: 2 in, 2 out]
              }
              frame "Relay", "Solenoid" {
                w252 = FALSE ("Visible")
                n141 = property on="Motor" class="Clust (strict)"("Visible"=w252) -> ()  [unwired: 2 in, 2 out]
                n142 = property on="Test Slider" class="Slide (strict)"("Visible"=w252) -> ()  [unwired: 2 in, 2 out]
                n143 = Search and Replace String(input string=w253, search string="/Value  **", replace string="/Direction") -> (result string=w259:string)  [unwired: 5 in, 3 out]
                n144 = property on="Test Ring" class="Ring (strict)"("Visible"=w252) -> ()  [unwired: 2 in, 2 out]
                n145 = call <vilib>:"NT Read String.vi"("Name"=w259) -> ("String"=w257:string)  [unwired: 9 in, 1 out]
                n146 = Equal?(x="Both directions", y=w257) -> (x = y?=w255:bool)
                n147 = Not(x=w255) -> (.not. x?=w256:bool)
                n148 = property on="Rev/Fwd" class="Clust (strict)"("Visible"=w255) -> ()  [unwired: 2 in, 2 out]
                n149 = property on="On/Off" class="Bool (strict)"("Visible"=w256, "Caption.Text"=w254) -> ()  [unwired: 2 in, 2 out]
              }
              frame "Compressor", "Digital Out" {
                w262 = FALSE ("Visible")
                # "Get direction and finish"
                n150 = property on="Motor" class="Clust (strict)"("Visible"=w262) -> ()  [unwired: 2 in, 2 out]
                n151 = property on="Test Slider" class="Slide (strict)"("Visible"=w262) -> ()  [unwired: 2 in, 2 out]
                n152 = property on="Test Ring" class="Ring (strict)"("Visible"=w262) -> ()  [unwired: 2 in, 2 out]
                n153 = property on="On/Off" class="Bool (strict)"("Visible"=TRUE, "Caption.Text"=w263) -> ()  [unwired: 2 in, 2 out]
                n154 = property on="Rev/Fwd" class="Clust (strict)"("Visible"=FALSE) -> ()  [unwired: 2 in, 2 out]
              }
              frame "Camera" {
                n155 = call <vilib>:"Get Last Path Segment.vi"("String in"=w270) -> ("String out"=w271:string)  [unwired: 10 in]
                n156 = property on="On/Off" class="Bool (strict)"("Visible"=FALSE) -> ()  [unwired: 2 in, 2 out]
                n157 = property on="Motor" class="Clust (strict)"("Visible"=FALSE) -> ()  [unwired: 2 in, 2 out]
                n158 = property on="Rev/Fwd" class="Clust (strict)"("Visible"=FALSE) -> ()  [unwired: 2 in, 2 out]
                n159 = case shown="\"Exposure Priority  **\"" w271 {
                  tunnel: w270 -> [w277 w286 w295 w304 w313 _ w319]
                  tunnel: w269 -> [w275 w283 w292 w301 w310 _ _]
                  frame "Size  **" {
                    n160 = Index Array(array=w275) -> (element=w274:cluster{string[]})  [unwired: 1 in]
                    n161 = call <vilib>:"NT Read String.vi"("Name"=w277) -> ("String"=w276:string)  [unwired: 9 in, 1 out]
                    n162 = Unbundle(w274) -> (w272:string[])
                    n163 = Match First String(2:w272, 3:w276) -> (0:w273:i32)  [unwired: 1 out]
                    n164 = property on="Test Ring" class="Ring (strict)"("Value"=w273, "Strings []"=w272) -> ()  [unwired: 2 in, 2 out]
                    n165 = property on="Test Ring" class="Ring (strict)"("Visible"=TRUE) -> ()  [unwired: 2 in, 2 out]
                    n166 = property on="Test Slider" class="Slide (strict)"("Visible"=FALSE) -> ()  [unwired: 2 in, 2 out]
                  }
                  frame "White Balance  **" {
                    n167 = Index Array(array=w283, index=1) -> (element=w284:cluster{string[]})
                    n168 = call <vilib>:"NT Read String.vi"("Name"=w286) -> ("String"=w285:string)  [unwired: 9 in, 1 out]
                    n169 = Unbundle(w284) -> (w281:string[])
                    n170 = Match First String(2:w281, 3:w285) -> (0:w280:i32)  [unwired: 1 out]
                    n171 = property on="Test Ring" class="Ring (strict)"("Value"=w280, "Strings []"=w281) -> ()  [unwired: 2 in, 2 out]
                    n172 = property on="Test Ring" class="Ring (strict)"("Visible"=TRUE) -> ()  [unwired: 2 in, 2 out]
                    n173 = property on="Test Slider" class="Slide (strict)"("Visible"=FALSE) -> ()  [unwired: 2 in, 2 out]
                  }
                  frame "Exposure  **" {
                    n174 = Index Array(array=w292, index=2) -> (element=w293:cluster{string[]})
                    n175 = call <vilib>:"NT Read String.vi"("Name"=w295) -> ("String"=w294:string)  [unwired: 9 in, 1 out]
                    n176 = Unbundle(w293) -> (w289:string[])
                    n177 = Match First String(2:w289, 3:w294) -> (0:w290:i32)  [unwired: 1 out]
                    n178 = property on="Test Ring" class="Ring (strict)"("Value"=w290, "Strings []"=w289) -> ()  [unwired: 2 in, 2 out]
                    n179 = property on="Test Ring" class="Ring (strict)"("Visible"=TRUE) -> ()  [unwired: 2 in, 2 out]
                    n180 = property on="Test Slider" class="Slide (strict)"("Visible"=FALSE) -> ()  [unwired: 2 in, 2 out]
                  }
                  frame "Exposure Priority  **" {
                    n181 = Index Array(array=w301, index=3) -> (element=w302:cluster{string[]})
                    n182 = call <vilib>:"NT Read String.vi"("Name"=w304) -> ("String"=w303:string)  [unwired: 9 in, 1 out]
                    n183 = Unbundle(w302) -> (w298:string[])
                    n184 = Match First String(2:w298, 3:w303) -> (0:w299:i32)  [unwired: 1 out]
                    n185 = property on="Test Ring" class="Ring (strict)"("Value"=w299, "Strings []"=w298) -> ()  [unwired: 2 in, 2 out]
                    n186 = property on="Test Ring" class="Ring (strict)"("Visible"=TRUE) -> ()  [unwired: 2 in, 2 out]
                    n187 = property on="Test Slider" class="Slide (strict)"("Visible"=FALSE) -> ()  [unwired: 2 in, 2 out]
                  }
                  frame "Color Enable  **" {
                    n188 = Index Array(array=w310, index=4) -> (element=w311:cluster{string[]})
                    n189 = call <vilib>:"NT Read String.vi"("Name"=w313) -> ("String"=w312:string)  [unwired: 9 in, 1 out]
                    n190 = Unbundle(w311) -> (w307:string[])
                    n191 = Match First String(2:w307, 3:w312) -> (0:w308:i32)  [unwired: 1 out]
                    n192 = property on="Test Ring" class="Ring (strict)"("Value"=w308, "Strings []"=w307) -> ()  [unwired: 2 in, 2 out]
                    n193 = property on="Test Ring" class="Ring (strict)"("Visible"=TRUE) -> ()  [unwired: 2 in, 2 out]
                    n194 = property on="Test Slider" class="Slide (strict)"("Visible"=FALSE) -> ()  [unwired: 2 in, 2 out]
                  }
                  frame Default {
                    n195 = property on="Test Ring" class="Ring (strict)"("Visible"=FALSE) -> ()  [unwired: 2 in, 2 out]
                    n196 = property on="Test Slider" class="Slide (strict)"("Visible"=FALSE) -> ()  [unwired: 2 in, 2 out]
                  }
                  frame "Brightness  **", "Color Level  **", "Compression  **", "FPS  **", "Sharpness  **" {
                    n197 = call <vilib>:"NT Read Number.vi"("Name"=w319) -> ("Numeric"=w318:dbl)  [unwired: 9 in, 1 out]
                    n198 = local write "Test Slider"(w318) -> ()
                    n199 = property on="Test Slider" class="Slide (strict)"("Visible"=TRUE, "Scale.Maximum"=100.0 ("Scale.Range:Maximum")) -> ()  [unwired: 2 in, 2 out]
                    n200 = property on="Test Ring" class="Ring (strict)"("Visible"=FALSE) -> ()  [unwired: 2 in, 2 out]
                  }
                }
              }
            }
            n201 = property on="Progress" class="Clust (strict)"("Visible"=FALSE) -> ()  [unwired: 2 in, 2 out]
          }
          event "Test Name": Mouse Enter {
            # "Populate the ring with the list of tests"
            n202 = event-data() -> ()  [unwired: 1 in, 1 out]
            n203 = call <vilib>:"NT Read String Array.vi"("Name"="TestMode/TestList") -> ("String Array"=w327:string[])  [unwired: 9 in, 1 out]
            n204 = Build Array (concatenate)("Select the test to run...", w327) -> (w326:string[])
            n205 = property on="Test Name" class="Ring (strict)"("Strings []"=w326) -> ()  [unwired: 2 in, 2 out]
          }
          event "Test Name": Value Change {
            w329 = FALSE ("Visible")
            # "Tell the robot the test name to run"
            n206 = event-data() -> ("NewVal"=w333:u16)  [unwired: 1 in]
            n207 = property on="Test Name" class="Ring (strict)"() -> ("Strings []"=w334:string[])  [unwired: 2 in, 2 out]
            n208 = local write "Progress"(T1 {"Test Progress"=0, "Test Progress Text"=""} ("Progress")) -> ()
            n209 = Index Array(array=w334, index=w333) -> (element=w332:string)
            n210 = call <vilib>:"NT Write String.vi"("String"=w332, "Name"="TestMode/TestName") -> ()  [unwired: 9 in, 1 out]
            n211 = property on="Progress" class="Clust (strict)"("Visible"=TRUE) -> ()  [unwired: 2 in, 2 out]
            n212 = property on="Motor" class="Clust (strict)"("Visible"=w329) -> ()  [unwired: 2 in, 2 out]
            n213 = property on="Test Slider" class="Slide (strict)"("Visible"=w329) -> ()  [unwired: 2 in, 2 out]
            n214 = property on="On/Off" class="Bool (strict)"("Visible"=w329) -> ()  [unwired: 2 in, 2 out]
            n215 = property on="Rev/Fwd" class="Clust (strict)"("Visible"=w329) -> ()  [unwired: 2 in, 2 out]
            n216 = property on="Test Ring" class="Ring (strict)"("Visible"=w329) -> ()  [unwired: 2 in, 2 out]
          }
          event "Listbox": Double Click {
            # "Shift clears all"
            # "Update symbols on the listbox"
            n217 = event-data() -> ("PlatMods.Shift"=w337:bool, "Row"=w339:i32)  [unwired: 1 in]
            n218 = case shown="True" w337 {
              tunnel: w339 -> [w343 _]
              tunnel: 1 -> [w342 _]
              frame False {
                n219 = property on="Listbox" class="LstBox (strict)"() -> ("Item Symbols"=w341:i32[])  [unwired: 2 in, 2 out]
                n220 = Replace Array Subset(array=w341, new element=w342, index=w343) -> (w340:i32[])
                n221 = property on="Listbox" class="LstBox (strict)"("Item Symbols"=w340) -> ()  [unwired: 2 in, 2 out]
              }
              frame True {
                w344 = 0 ("Top Row")
                n222 = property on="Listbox" class="LstBox (strict)"() -> ("Number of Rows"=w346:u32)  [unwired: 2 in, 2 out]
                n223 = Initialize Array(0, w346) -> (w345:i32[])
                n224 = property on="Listbox" class="LstBox (strict)"("Top Row"=w344, "Value"=w344, "Item Symbols"=w345) -> ()  [unwired: 2 in, 2 out]
              }
            }
          }
          event "Listbox": Key Down {
            # "Update symbols on the listbox\nLeft and right keys check and uncheck"
            n225 = event-data() -> ("VKey"=w350:T24)  [unwired: 1 in]
            n226 = case shown="\"Left\", \"Right\"" w350 {
              selector: w350 -> [w355 _]
              tunnel: eventvkey."Left" ("VKey") -> [w353 _]
              frame "Left", "Right" {
                n227 = Equal?(x=w353, y=w355) -> (x = y?=w354:bool)
                n228 = Select(t=0, s=w354, f=1) -> (s? t:f=w356:i32)
                n229 = property on="Listbox" class="LstBox (strict)"() -> ("Item Symbols"=w359:i32[])  [unwired: 2 in, 2 out]
                n230 = Replace Array Subset(array=w359, new element=w356, index="Listbox") -> (w358:i32[])
                n231 = property on="Listbox" class="LstBox (strict)"("Item Symbols"=w358) -> ()  [unwired: 2 in, 2 out]
              }
              frame Default {
              }
            }
          }
          event #6 (no event record) {
            # "Show or hide the cluster of controls, store in ini file"
            n232 = event-data() -> ("NewVal"=w363)  [unwired: 1 in]
            n233 = case shown="False" w363 {
              tunnel: w362 -> [w372 _]
              tunnel: [w365 w383] -> w361
              tunnel: w360 -> [w364 w383]
              frame False {
                w379 = "Camera"
                n234 = Index Array(array=w372) -> (element=w375:cluster{string[]})  [unwired: 1 in]
                n235 = local read item#-1() -> (w371)
                n236 = Unbundle(w371) -> (w370, w369, w373)
                n237 = Unbundle(w375) -> (w374:string[])
                n238 = Index Array(array=w374, index=w373) -> (element=w368:string)
                n239 = call-poly <vilib>:"Write Key.vi"("section"=w379, "value"=w368, "key"="Size", "refnum"=w364) -> ("refnum out"=w381:T27)  [unwired: 2 in, 5 out]
                n240 = call-poly <vilib>:"Write Key.vi"("section"=w379, "value"=w370, "key"="FrameRate", "refnum"=w381) -> ("refnum out"=w380:T27)  [unwired: 1 in, 6 out]
                n241 = call-poly <vilib>:"Write Key.vi"("section"=w379, "value"=w369, "key"="Compression", "refnum"=w380) -> ("refnum out"=w366:T27)  [unwired: 1 in, 6 out]
                n242 = local write item#-1(FALSE ("Visible")) -> ()
                n243 = call <vilib>:"Close Config Data.vi"("refnum"=w366) -> ("file path"=w367:path)  [unwired: 2 in, 8 out]
                n244 = call <vilib>:"Open Config Data.vi"("configuration file path"=w367) -> ("refnum"=w365:T27)  [unwired: 8 in, 2 out]
              }
              frame True {
                (unwired) TRUE ("Visible")
              }
            }
          }
          event #7 (no event record) {
            # "Update summary string when any elements of DB camera change"
            n245 = event-data() -> ("NewVal"=w394)  [unwired: 1 in]
            n246 = Index Array(array=w391) -> (element=w390:cluster{string[]})  [unwired: 1 in]
            n247 = Unbundle(w394) -> (w386, w385, w388)
            n248 = Unbundle(w390) -> (w389:string[])
            n249 = Index Array(array=w389, index=w388) -> (element=w387:string)
            n250 = Format Into String(format string="%s   %dfps   %d%%", w387, w386, w385) -> (resulting string=w392:string)  [unwired: 2 in, 1 out]
            n251 = Build Array(w392) -> ()  [unwired: 1 out]
          }
          event "Motor.Enable": Value Change {
            # "When the test mode otor enable helper is set, update that\ntree row item's value"
            n252 = event-data() -> ("NewVal"=w400:bool)  [unwired: 1 in]
            n253 = Unbundle("Motor") -> ("Value"=w399:dbl)  [unwired: 1 out]
            n254 = Select(t=w399, s=w400, f=0.0) -> (s? t:f=w397:dbl)
            n255 = call <vilib>:"NT Write Number.vi"("Numeric"=w397, "Name"=w396) -> ()  [unwired: 9 in, 1 out]
          }
          event "Test Slider": Value Change {
            # "When the test mode slider helper is set, update that\ntree row item's value"
            n256 = event-data() -> ("NewVal"=w403:dbl)  [unwired: 1 in]
            n257 = call <vilib>:"NT Write Number.vi"("Numeric"=w403, "Name"=w404) -> ()  [unwired: 9 in, 1 out]
          }
          event "On/Off": Value Change {
            # "When the test mode on/off helper value is set, update that\ntree row item's value"
            n258 = event-data() -> ("NewVal"=w408:bool)  [unwired: 1 in]
            n259 = Boolean To (0,1)(Boolean=w408) -> (0, 1=w407:i16)
            n260 = call <vilib>:"NT Write Number.vi"("Numeric"=w407, "Name"=w406) -> ()  [unwired: 9 in, 1 out]
          }
          event "Rev/Fwd": Value Change {
            # "When the test mode helper value for relays is set, update that\ntree row item's value"
            n261 = event-data() -> ("NewVal.Forward"=w416:bool, "NewVal.Reverse"=w415:bool)  [unwired: 1 in]
            n262 = Boolean To (0,1)(Boolean=w416) -> (0, 1=w412:i16)
            n263 = Boolean To (0,1)(Boolean=w415) -> (0, 1=w414:i16)
            n264 = Negate(x=w414) -> (-x=w413:i16)
            n265 = Add(x=w412, y=w413) -> (x+y=w411:i16)
            n266 = call <vilib>:"NT Write Number.vi"("Numeric"=w411, "Name"=w410) -> ()  [unwired: 9 in, 1 out]
          }
          event "Test Ring": Value Change {
            # "When a test mode helper value is selected from the ring,\nset the tree item's variable to the string value"
            n267 = event-data() -> ("NewVal"=w420:u16)  [unwired: 1 in]
            n268 = property on="Test Ring" class="Ring (strict)"() -> ("Strings []"=w421:string[])  [unwired: 2 in, 2 out]
            n269 = Index Array(array=w421, index=w420) -> (element=w419:string)
            n270 = call <vilib>:"NT Write String.vi"("String"=w419, "Name"=w418) -> ()  [unwired: 9 in, 1 out]
          }
          event "Rec Mode": Value Change {
            # "Update globals for recording mode and path to read log from.\nClear when logging and let NetworkTables set path for vision to\nuse."
            n271 = event-data() -> ("NewVal"=w431:enum32{"Stop", "Record", "Playback"})  [unwired: 1 in]
            n272 = case shown="\"Stop\", \"Record\"" w431 {
              tunnel: w430 -> [_ w433 w441]
              tunnel: [_ _ w440] -> w427
              tunnel: [_ _ w439] -> _
              tunnel: w425 -> [_ _ w437]
              tunnel: cluster{i32, i32} {-250, 170} -> [_ _ w436]
              tunnel: [_ _ T25 {"Image Size"=TRUE, "Image Type"=TRUE, "Pixel Value"=TRUE, "ROI Information"=TRUE, "Zoom Factor"=FALSE} ("Image Information Shown:All Elements")] -> w423
              tunnel: [_ _ TRUE ("Zoom Factor")] -> w422
              frame Default {
              }
              frame "Stop", "Record" {
                # "Place Window too"
                n273 = invoke class="VI" method="FP.Close"(reference=w433) -> (reference out=w432:refnum<vi>)  [unwired: 2 in, 2 out]
                n274 = invoke class="VI" method="Abort VI"(reference=w432) -> ()  [unwired: 2 in, 3 out]
              }
              frame "Playback" {
                n275 = call "Open Playback Panel.vi"("Offset"=w436, "DB VI Ref"=w437, "Playback in"=w441) -> ("Playback out"=w438:refnum<vi>)  [unwired: 8 in]
                n276 = register-events(w438) -> (reference out=w440:refnum<event-registration>, error out=w439:errorcluster)  [unwired: 2 in]
              }
            }
            n277 = global write "WPI_DashboardLogging Global.vi" "Logging Filename"(path "") -> ()
            n278 = global write "WPI_DashboardLogging Global.vi" "Recording"(w431) -> ()
            n279 = property on="Camera Image" class="ImageControl"("Image Information Shown"=w423, "Image Information Visible"=w422) -> ()  [unwired: 2 in, 2 out]
            n280 = call <vilib>:"WPI_DashboardNT Log FieldName Cache.vi"("Operation"=enum16{"Lookup/Add", "Index", "Clear"}."Clear") -> ()  [unwired: 8 in, 3 out]
          }
          event Panel Close {
            w442 = enum32{"Stop", "Record", "Playback"}."Stop" ("Rec Mode")
            # "Playback window has been closed, abort"
            n281 = event-data() -> ()  [unwired: 1 in, 4 out]
            n282 = local write "Rec Mode"(w442) -> ()
            n283 = global write "WPI_DashboardLogging Global.vi" "Recording"(w442) -> ()
          }
          event Panel Close {
            # "Abort playback window and ourself"
            n284 = event-data() -> ()  [unwired: 1 in, 4 out]
            n285 = invoke class="VI" method="FP.Close"(reference=w447) -> (reference out=w446:refnum<vi>)  [unwired: 2 in, 2 out]
            n286 = invoke class="VI" method="Abort VI"(reference=w446) -> (error out=w445:errorcluster)  [unwired: 2 in, 2 out]
            n287 = invoke class="VI" method="Abort VI"(error in=w445) -> ()  [unwired: 2 in, 3 out]
          }
          event "Vision": Value Change {
            # "Enable/Disable Compression slider.\nHW USB is hard-coded into the camera"
            n288 = event-data() -> ("NewVal"=w453:u16)  [unwired: 1 in]
            n289 = Equal?(x=w453, y=u32 2 ("milliseconds to wait")) -> (x = y?=w451:bool)
            n290 = Select(t=T26."Disabled and Grayed Out" ("Disabled"), s=w451, f=T26."Enabled" ("Disabled")) -> (s? t:f=w448:T26)
          }
        }
      }
      n291 = property on="On/Off" class="Bool (strict)"("Visible"=w150) -> ()  [unwired: 2 in, 2 out]
      n292 = property on="Motor" class="Clust (strict)"("Visible"=w150) -> ()  [unwired: 2 in, 2 out]
      n293 = property on="Progress" class="Clust (strict)"("Visible"=w150) -> ()  [unwired: 2 in, 2 out]
      n294 = property on="Test Ring" class="Ring (strict)"("Visible"=w150) -> ()  [unwired: 2 in, 2 out]
      n295 = property on="Rev/Fwd" class="Clust (strict)"("Visible"=w150) -> ()  [unwired: 2 in, 2 out]
      n296 = local write item#-1(w150) -> ()
      n297 = global write "WPI_DashboardLogging Global.vi" "Recording"(w149) -> ()
      n298 = local write "Rec Mode"(w149) -> ()
    }
    frame Enabled {
      # "More Unneeded Stuff (Hidden and Disabled)"
    }
  }
